vi "SiosIfmStartBlock.vi"(1 "Block Length":i32, 2 "Device Number":i32) -> (0 "Success":i32)   [LabVIEW 2009]
uses:
  siosifm.dll
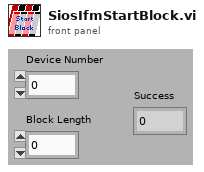
[diagram p1: front panel]
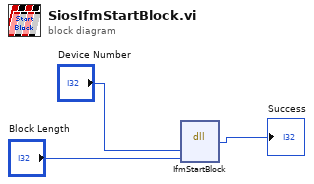
[diagram p0: block diagram]
diagram:
  n1 = dll-call lib="C:/WORK/Artem/RE-10/SIOS_IfmDLL/siosifm.dll" fn="IfmStartBlock"("devNumber"="Device Number", "blockLen"="Block Length") -> ("success"=→"Success":i32)  [unwired: 5 in, 2 out]
